vi "ToIScan.vi"(11 "OfficeTron3000.lvlib:OfficeTron3000.lvclass":refnum<class "OfficeTron3000.lvclass">) -> (2 "OfficeTron3000.lvlib:OT3IScan.lvclass":refnum<class "OT3IScan.lvclass">)   [LabVIEW 2018, in "OfficeTron3000.lvlib" / "OfficeTron3000.lvclass"]
uses:
  OfficeTron3000.lvclass
  OT3IScan/OT3IScan.lvclass
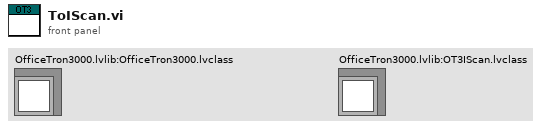
[diagram p1: front panel]
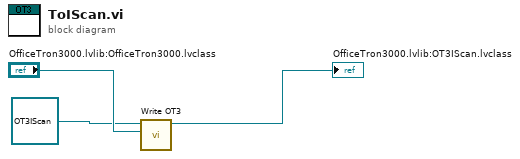
[diagram p0: block diagram]
diagram:
  n1 = call "Write OT3.vi"("OT3"="OfficeTron3000.lvlib:OfficeTron3000.lvclass", "OT3IScan in"=refnum<class "OT3IScan.lvclass"> refnum) -> ("OT3IScan out"=→"OfficeTron3000.lvlib:OT3IScan.lvclass":refnum<class "OT3IScan.lvclass">)  [unwired: 9 in]
